vi "test-Counter.vi"() -> ()   [LabVIEW 2017]
uses:
  Signal/_Number Count Down(Array).vi
  Signal/_Number Count Down(Element).vi
  Signal/_Number Count Down(Array).vi/9de0e42d-c65c-4cbc-a92d-661ac054e2ac.vi
panel:
  out "left 3":i64[](array[numeric])
  out "left 2":i64
  out "left":i64
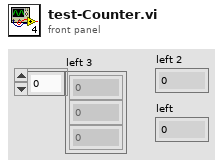
[diagram p1: front panel]
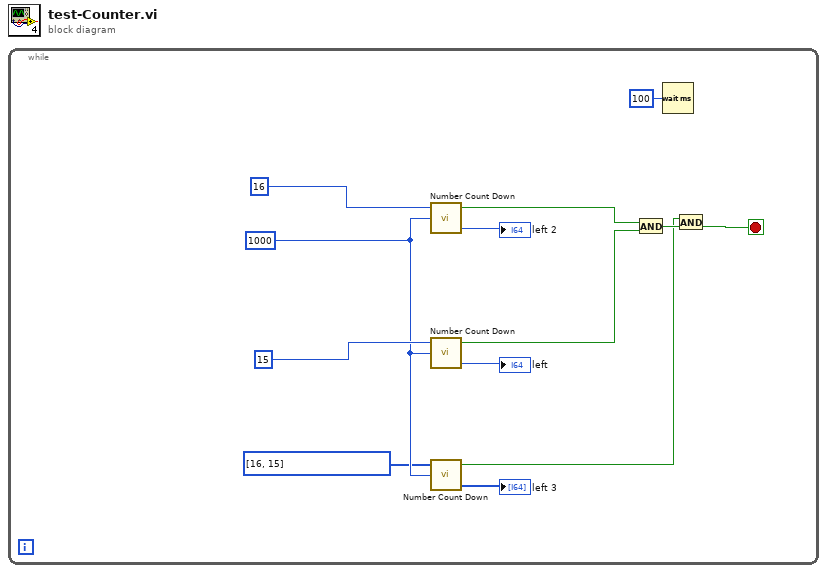
[diagram p0: block diagram]
diagram:
  n1 = while {
    stop <- w2 stop-if-true
    w5 = i64 1000 ("threasholds")
    n2 = call-poly "Number Count Down.vi"("number"=16 ("Numeric 2"), "threashold"=w5) -> ("reach?"=w11:bool, "left"=→"left 2":i64)  [unwired: 6 in]
    n3 = call-poly "Number Count Down.vi"("number"=15 ("Numeric"), "threashold"=w5) -> ("reach?"=w10:bool, "left"=→"left":i64)  [unwired: 6 in]
    n4 = call-poly "Number Count Down.vi"("fixed size array"=i32[] [16, 15], "threashold"=w5) -> ("reach?"=w1:bool, "left"=→"left 3":i64[])  [unwired: 6 in]
    n5 = And(x=w11, y=w10) -> (x .and. y?=w9:bool)
    n6 = Wait (ms)(milliseconds to wait=u32 100) -> ()  [unwired: 1 out]
    n7 = And(x=w1, y=w9) -> (x .and. y?=w2:bool)
  }
